vi "Activate Window then Click Position.vi"   [LabVIEW 2022 SP3]
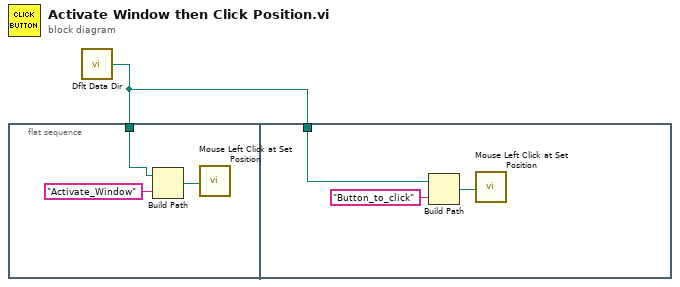
[diagram p0: block diagram]
diagram:
  n1 = flat-sequence {
    tunnel: w1 -> [w2]
    tunnel: w1 -> [w5]
    frame #0 {
      n2 = Build Path(base path=w2, name or relative path="Activate_Window") -> (appended path=w3:path)
      n3 = call "Mouse Left Click at Set Position.vi"("Click position file path"=w3) -> ()  [unwired: 1 out]
    }
    frame #1 {
      n4 = Build Path(base path=w5, name or relative path="Button_to_click") -> (appended path=w7:path)
      n5 = call "Mouse Left Click at Set Position.vi"("Click position file path"=w7) -> ()  [unwired: 1 out]
    }
  }
  n6 = call <vilib>:"Dflt Data Dir.vi"() -> ("App:Default Data Directory"=w1:path)
